vi "About Screen.vi"(10 "About Config File Name":string) -> ()   [LabVIEW 2013, in "About Screen Library.lvlib"]
uses:
  About Screen Library.lvlib
  <vilib>/Platform/browser.llb/Open URL in Default Browser (string).vi
panel:
  in  "Hyperlink":bool
  in  "Close Screen":bool
  out "Logo (80 x 80)":picture
  out "About Text":string
  out "Banner (720 x 80)":picture
  # "Click to continue"
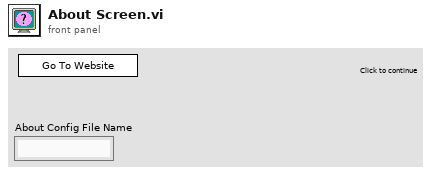
[diagram p1: front panel]
types:
  T1 = typedef "About Screen Library.lvlib/Configuration Data.ctl" = cluster{"Window Title":string, "About Text":string, "Include Hyperlink?":bool, "Hyperlink Path":string, "Logo (80 x 80)":picture, "Banner (720 x 80)":picture, "Background Color":u32}
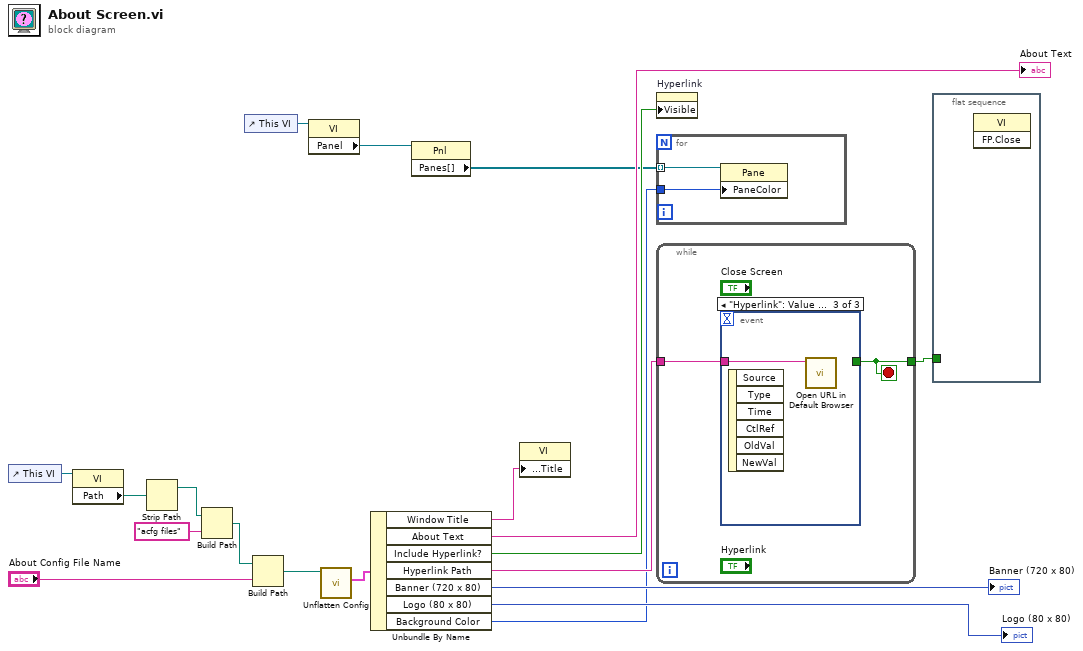
[diagram p0: block diagram]
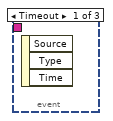
[diagram p2: hidden frame]
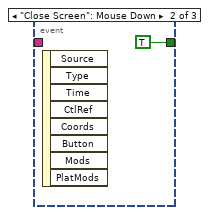
[diagram p3: hidden frame]
diagram:
  n1 = control-ref of="This VI"() -> (w8:refnum<vi>)
  n2 = property class="VI"(reference=w8) -> ("Path"=w7:path)  [unwired: 1 in, 2 out]
  n3 = Strip Path(path=w7) -> (stripped path=w6:path)  [unwired: 1 out]
  n4 = Build Path(base path=w6, name or relative path="acfg files") -> (appended path=w5:path)
  n5 = control-ref of="This VI"() -> (w13:refnum<vi>)
  n6 = Build Path(base path=w5, name or relative path="About Config File Name") -> (appended path=w2:path)
  n7 = property class="VI"(reference=w13) -> ("Panel"=w12:refnum<vi>)  [unwired: 1 in, 2 out]
  n8 = call "Unflatten Config.vi"("About Configuration File"=w2) -> ("About Configuration"=w19:T1)  [unwired: 9 in, 1 out]
  n9 = Unbundle By Name(w19) -> ("Window Title"=w1:string, "About Text"=→"About Text":string, "Include Hyperlink?"=w17:bool, "Hyperlink Path"=w16:string, "Banner (720 x 80)"=→"Banner (720 x 80)":picture, "Logo (80 x 80)"=→"Logo (80 x 80)":picture, "Background Color"=w10:u32)
  n10 = property class="Pnl"(reference=w12) -> ("Panes[]"=w11:refnum<vi>[])  [unwired: 1 in, 2 out]
  n11 = property class="VI"("Front Panel.Title"=w1) -> ()  [unwired: 2 in, 2 out]
  n12 = property on="Hyperlink" class="Bool"("Visible"=w17) -> ()  [unwired: 2 in, 2 out]
  n13 = for {
    tunnel: w11 -> [w21] mode=indexing
    tunnel: w10 -> [w20]
    n14 = property class="Pane"(reference=w21, "PaneColor"=w20) -> ()  [unwired: 1 in, 2 out]
  }
  n15 = while {
    tunnel: w16 -> [w23]
    tunnel: [w22] -> w9
    stop <- w22 stop-if-true
    n16 = event shown="[2] \"Hyperlink\": Value Change" {
      selector: _ -> [_ _ _]
      dyn-events: _ -> [_ _ _]
      timeout: _ -> [_ _ _]
      tunnel: [_ TRUE _] -> w22
      tunnel: w23 -> [_ _ w25]
      event Timeout {
        n17 = event-data() -> ()  [unwired: 1 in, 3 out]
      }
      event "Close Screen": Mouse Down {
        n18 = event-data() -> ()  [unwired: 1 in, 8 out]
      }
      event "Hyperlink": Value Change {
        n19 = event-data() -> ()  [unwired: 1 in, 6 out]
        n20 = call-poly <vilib>:"Open URL in Default Browser.vi"("URL"=w25) -> ()  [unwired: 5 in, 2 out]
      }
    }
  }
  n21 = flat-sequence {
    tunnel: w9 -> [_]
    frame #0 {
      n22 = invoke class="VI" method="FP.Close"() -> ()  [unwired: 3 in, 3 out]
    }
  }
